vi "Write PC Beamage.vi"(8 "error in":errorcluster, 10 "command":string="*ver") -> (0 "error out":errorcluster)   [LabVIEW 2009]
uses:
  BeamageNP.dll
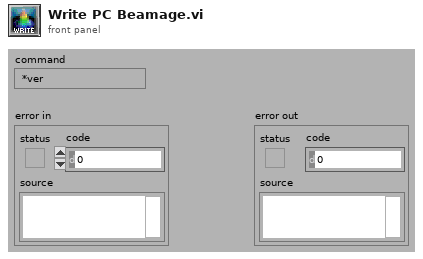
[diagram p1: front panel]
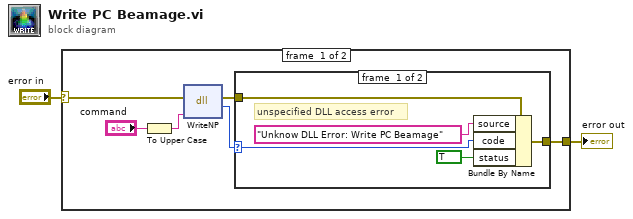
[diagram p0: block diagram]
diagram:
  n1 = case shown="No Error" "error in" {
    selector: "error in" -> [w6 w15]
    tunnel: [w4 w15] -> w1
    frame #0 {
      n2 = To Upper Case(1:"command") -> (0:w7:string)
      n3 = dll-call lib="S:/LabView Files/Beamage 3.0/BeamageNP.dll" fn="WriteNP"(error in=w6, "command"=w7) -> (error out=w3:errorcluster, "success"=w5:i32)  [unwired: 3 in, 1 out]
      n4 = case shown="1" w5 {
        selector: w5 -> [w11 _]
        tunnel: [w9 w14] -> w4
        tunnel: w3 -> [w13 w14]
        frame #0 {
          # "unspecified DLL access error"
          n5 = Bundle By Name(cluster=w13, "source"="Unknow DLL Error: Write PC Beamage", "code"=w11, "status"=TRUE) -> (w9:errorcluster)
        }
        frame #1 {
          # "if a 1 was returned no error"
        }
      }
    }
    frame #1 {
    }
  }
  "error out" <- w1
